vi "Data Logger Error Handling.vi"(3 "error in":errorcluster, 4 "Enum":enum16{"Main", "Event", "Config"}(ring)) -> (9 "error out":errorcluster)   [LabVIEW 2014]
uses:
  <vilib>/Utility/error.llb/DialogType.ctl
  <vilib>/Utility/file.llb/Read From Spreadsheet File (string).vi
panel:
  out "code out 3":i32 format="%0.0f"
  out "code out":i32 format="%0.0f"
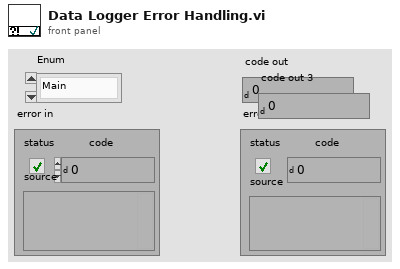
[diagram p1: front panel]
types:
  T1 = enum16{"Config File", "Image File", "Word Template", "Release Note", "Help HTML", "Help Word", "Error List", "Excel Template", "CSV Template"}
  T2 = typedef "DialogType.ctl" = u16
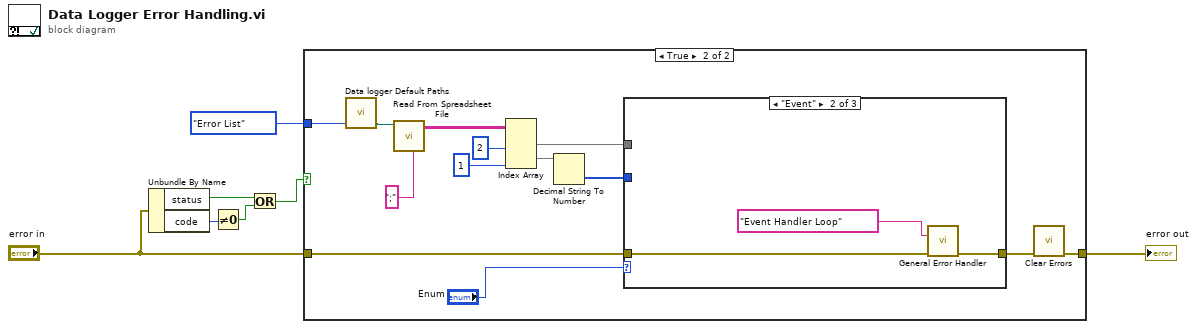
[diagram p0: block diagram]
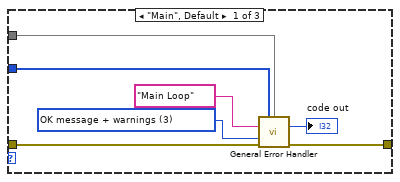
[diagram p3: hidden frame]
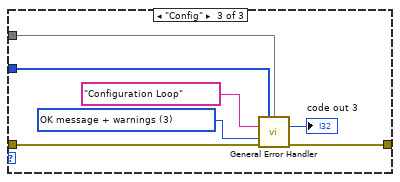
[diagram p4: hidden frame]
diagram:
  n1 = Unbundle By Name("error in") -> ("status"=w3:bool, "code"=w5:i32)
  n2 = Not Equal To 0?(x=w5) -> (x != 0?=w4:bool)
  n3 = Or(x=w3, y=w4) -> (x .or. y?=w2:bool)
  n4 = case shown="True" w2 {
    tunnel: [w8 w13] -> w7
    tunnel: "error in" -> [w8 w12]
    tunnel: T1."Error List" ("Path Type") -> [_ w10]
    frame False {
    }
    frame True {
      n5 = call "Data logger Default Paths.vi"("Path Type"=w10) -> ("Path"=w21:path)  [unwired: 4 in]
      n6 = call-poly <vilib>:"Read From Spreadsheet File.vi"("delimiter (\\t)"=";" ("delimiter (\\t)"), "file path (dialog if empty)"=w21) -> ("all rows"=w20:string[][])  [unwired: 5 in, 4 out]
      n7 = Index Array(array=w20, index (col) #1=2 ("disabled index (col)"), index (col) #2=1 ("index (col)")) -> (element #1=w17:string[], element #2=w16:string[])  [unwired: 2 in]
      n8 = Decimal String To Number(string=w16) -> (number=w15:i32[])  [unwired: 2 in, 1 out]
      n9 = case shown="\"Event\"" "Enum" {
        tunnel: w17 -> [w28 _ w38]
        tunnel: w15 -> [w27 _ w37]
        tunnel: [w24 w31 w34] -> w14
        tunnel: w12 -> [w23 w30 w33]
        frame "Main", Default {
          w25 = T2 3 items=["no dialog", "OK message", "continue or stop message", "OK message + warnings", "continue/stop + warnings"] ("type of dialog (OK msg:1)")
          n10 = call <vilib>:"General Error Handler.vi"("[user-defined codes]"=w27, "[user-defined descriptions]"=w28, "[error source] (\" \")"="Main Loop" ("[error source] (\" \")"), "type of dialog (OK msg:1)"=w25, "error in (no error)"=w23) -> ("code out"=→"code out":i32, "error out"=w24:errorcluster)  [unwired: 6 in, 3 out]
        }
        frame "Event" {
          n11 = call <vilib>:"General Error Handler.vi"("[error source] (\" \")"="Event Handler Loop" ("[error source] (\" \")"), "error in (no error)"=w30) -> ("error out"=w31:errorcluster)  [unwired: 9 in, 4 out]
        }
        frame "Config" {
          w35 = T2 3 items=["no dialog", "OK message", "continue or stop message", "OK message + warnings", "continue/stop + warnings"] ("type of dialog (OK msg:1)")
          n12 = call <vilib>:"General Error Handler.vi"("[user-defined codes]"=w37, "[user-defined descriptions]"=w38, "[error source] (\" \")"="Configuration Loop" ("[error source] (\" \")"), "type of dialog (OK msg:1)"=w35, "error in (no error)"=w33) -> ("code out"=→"code out 3":i32, "error out"=w34:errorcluster)  [unwired: 6 in, 3 out]
        }
      }
      n13 = call <vilib>:"Clear Errors.vi"("error in (no error)"=w14) -> ("error out"=w13:errorcluster)  [unwired: 5 in, 1 out]
    }
  }
  "error out" <- w7
